vi "Pathing V2.vi"() -> ()   [LabVIEW 2017]
uses:
  <vilib>/robotics/Navigation/shared/WorldMap/OccupancyGridWorldMap/NI_Robotics_OccupancyGridWorldMap.lvclass
  040-typeDefs/Position.ctl
  <vilib>/Analysis/NI_AALPro.lvlib
panel:
  out "Numeric":i32=24
  in  "Position":T1={"X Pos"=300.0, "Y Pos"=0.0, "Bearing"=0.0}
  in  "Initialpos":cluster{dbl, dbl, dbl}={300.0, 0.0, 0.0}
  out "path":cluster{"X":i32, "Y":i32}[](array[cluster])=[{"X"=3, "Y"=0}, {"X"=3, "Y"=1}, {"X"=3, "Y"=2}, {"X"=3, "Y"=3}, {"X"=3, "Y"=4}, {"X"=3, "Y"=5}, {"X"=3, "Y"=6}]
  out "XY Graph 3":cluster{dbl[], dbl[]}(graph)={[0.0, 0.0, 0.0, 0.0, 0.0, 0.0], [100.0, 200.0, 300.0, 400.0, 500.0, 600.0]}
  in  "Robot Relative Position":cluster{"PosX":dbl, "PosY":dbl}={"PosX"=-300.0, "PosY"=50.0}
  in  "map reference in 2":refnum<data-value>
  in  "map reference in":refnum<data-value>
  in  "stop 2":bool
  out "output cluster":cluster{"PosX":dbl, "PosY":dbl}
  in  "Resolution":dbl=100.0
  out "Intensity Graph":dbl[][](graph)
  out "XY Graph 2":cluster{dbl[], dbl[]}(graph)
  out "Final X, Y, BEARING":cluster{dbl, dbl, dbl}={245.38756896666968, 124.45046063453532, -26.464846153846153}
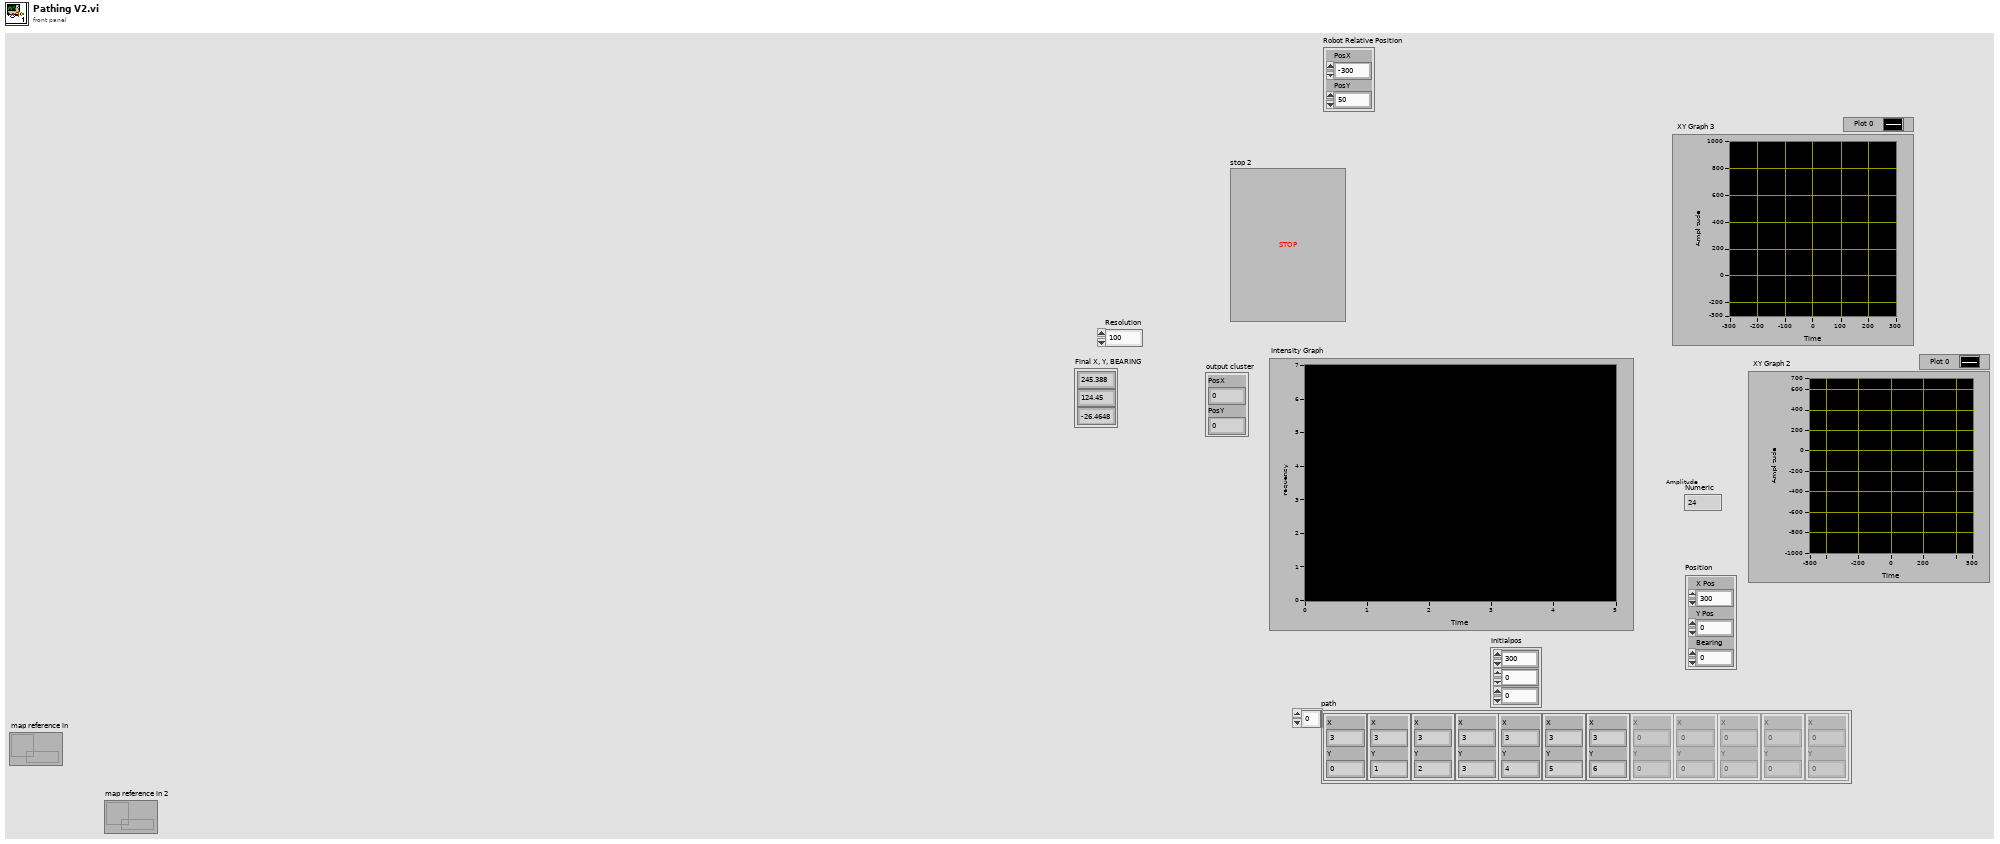
[diagram p1: front panel]
types:
  T1 = typedef "Position.ctl" = cluster{"X Pos":dbl, "Y Pos":dbl, "Bearing":dbl}
  T2 = typedef "LidarPoint.ctl" = cluster{"X":dbl, "Y":dbl}
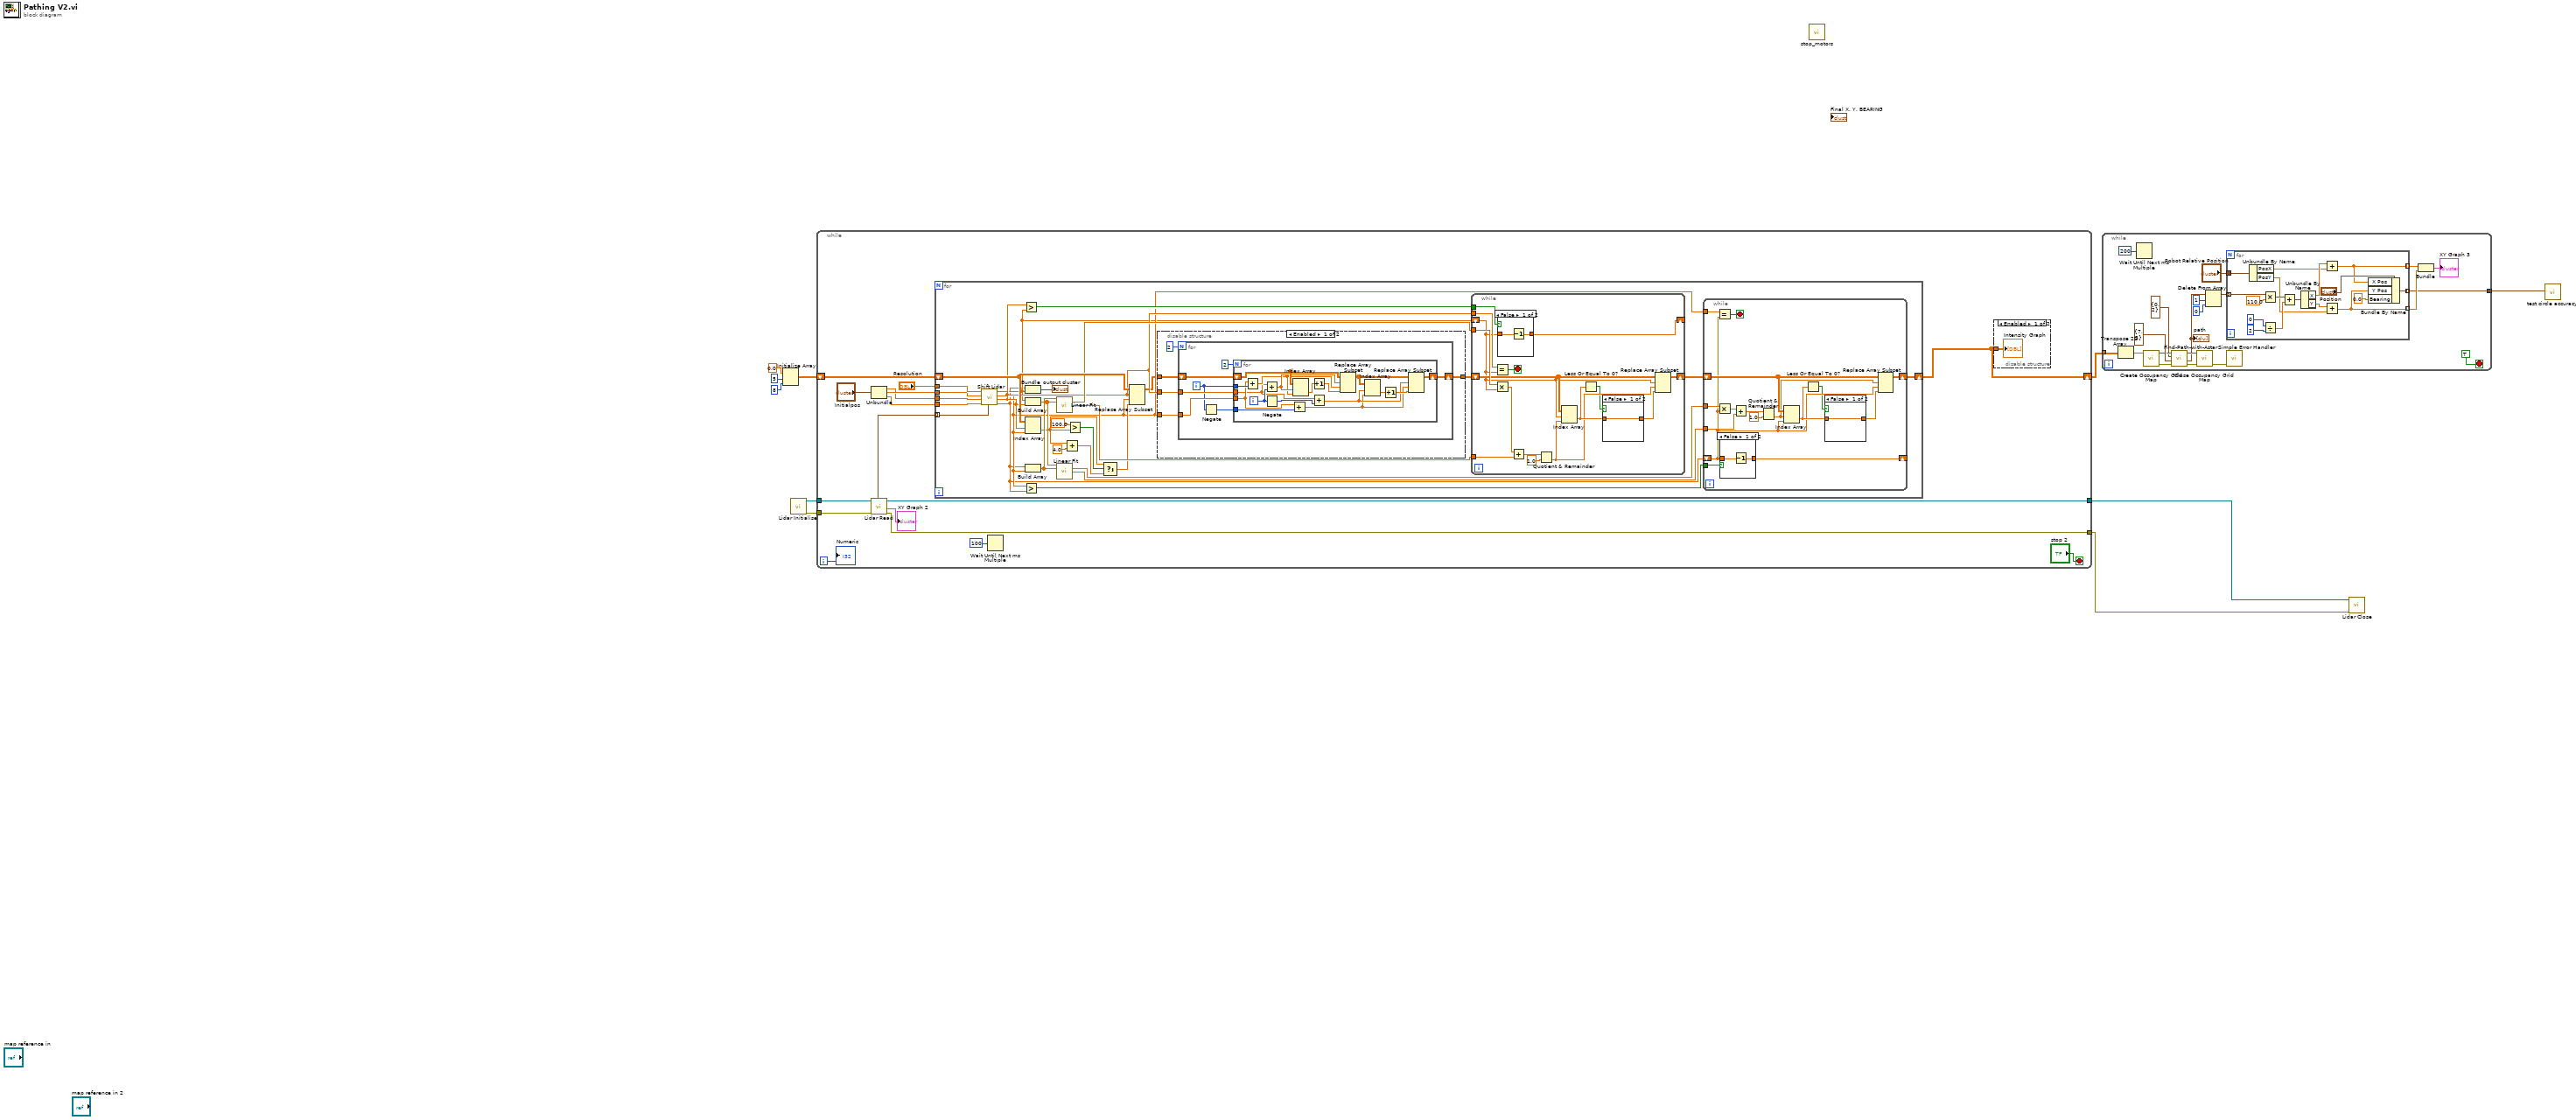
[diagram p0: block diagram]
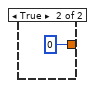
[diagram p4: hidden frame]
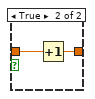
[diagram p5: hidden frame]
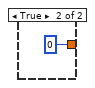
[diagram p6: hidden frame]
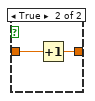
[diagram p7: hidden frame]
diagram:
  n1 = Initialize Array(0.0 ("element"), 5 ("dimension size"), 8 ("dimension size")) -> (w4:dbl[][])
  n2 = call "Lidar Initialise.vi"() -> ("error out"=w10:errorcluster, "VISA resource name out"=w3:refnum<visa-resource-name>)  [unwired: 10 in]
  n3 = while {
    tunnel: w3 -> [w26]
    tunnel: w10 -> [w25]
    tunnel: [w24] -> w9
    tunnel: [w23] -> w8
    shift-right: [w18] -> w2
    shift-left: w4 -> [w20]
    i -> [w11]
    stop <- "stop 2" stop-if-true
    n4 = Unbundle("Initialpos") -> (w13:dbl, w14:dbl, w12:dbl)
    n5 = call "Lidar Read.vi"("error in (no error)"=w25, "VISA resource name"=w26) -> ("error out"=w23:errorcluster, "Visual Out"=→"XY Graph 2":cluster{dbl[], dbl[]}, "VISA resource name out"=w24:refnum<visa-resource-name>, "XYflipped"=w19:T2[])  [unwired: 2 in, 3 out]
    n6 = for {
      tunnel: w14 -> [w54]
      tunnel: w13 -> [w49]
      tunnel: "Resolution" -> [w56]
      tunnel: w19 -> [w55] mode=indexing
      shift-right: [w34] -> w18
      shift-left: w20 -> [w53]
      tunnel: w12 -> [w33]
      n7 = call "Shift Lidar.vi"("XY"=w55, "Angle"=w33, "X position"=w49, "Y position"=w54, "Resolution"=w56) -> ("PosY"=w30:dbl, "Shifted X"=w36:dbl, "Shifted Y"=w35:dbl, "PosX"=w31:dbl)  [unwired: 3 in]
      n8 = Greater?(x=w36, y=w31) -> (0:w50:bool)
      n9 = Greater?(x=w35, y=w30) -> (0:w46:bool)
      n10 = Bundle("PosY"=w30, "PosX"=w31) -> (→"output cluster":cluster{"PosY":dbl, "PosX":dbl})  [unwired: 1 in]
      n11 = Build Array(w31, w36) -> (w44:dbl[])
      n12 = Index Array(array=w53, index (row)=w36, index (col)=w35) -> (element=w37:dbl)
      n13 = Build Array(w30, w35) -> (w45:dbl[])
      n14 = call <vilib>:"Linear Fit.vi"("Y"=w45, "X"=w44) -> ("slope"=w52:dbl, "intercept"=w51:dbl)  [unwired: 9 in, 3 out]
      n15 = call <vilib>:"Linear Fit.vi"("Y"=w44, "X"=w45) -> ("slope"=w43:dbl, "intercept"=w42:dbl)  [unwired: 9 in, 3 out]
      n16 = Add(x=w37, y=4.0) -> (x+y=w38:dbl)
      n17 = Greater?(x=100.0, y=w37) -> (0:w40:bool)
      n18 = Select(t=w37, s=w40, f=w38) -> (s? t:f=w41:dbl)
      n19 = Replace Array Subset(array=w53, new element=w41, index (row)=w36, index (col)=w35) -> (w29:dbl[][])
      n20 = disable-structure shown="Enabled" {
        disable-tunnel: w36 -> [w60 _]
        disable-tunnel: w35 -> [w59 _]
        disable-tunnel: w29 -> [w58 _]
        disable-tunnel: [w57 _] -> w28
        frame Enabled {
          n21 = for {
            N: 2 -> [_]
            tunnel: w60 -> [w66]
            tunnel: w59 -> [w64]
            shift-right: [w67] -> w57
            shift-left: w58 -> [w68]
            i -> [w63]
            n22 = Negate(x=w63) -> (-x=w62:i32)
            n23 = for {
              N: 2 -> [_]
              tunnel: w66 -> [w73]
              tunnel: w64 -> [w74]
              tunnel: w63 -> [w78]
              tunnel: w62 -> [w72]
              shift-right: [w81] -> w67
              shift-left: w68 -> [w83]
              i -> [w79]
              n24 = Add(x=w74, y=w78) -> (x+y=w75:dbl)
              n25 = Add(x=w73, y=w79) -> (x+y=w76:dbl)
              n26 = Negate(x=w79) -> (-x=w71:i32)
              n27 = Add(x=w74, y=w72) -> (x+y=w69:dbl)
              n28 = Index Array(array=w83, index (row)=w76, index (col)=w75) -> (element=w85:dbl)
              n29 = Increment(x=w85) -> (x+1=w77:dbl)
              n30 = Add(x=w73, y=w71) -> (x+y=w70:dbl)
              n31 = Replace Array Subset(array=w83, new element=w77, index (row)=w76, index (col)=w75) -> (w82:dbl[][])
              n32 = Index Array(array=w82, index (row)=w70, index (col)=w69) -> (element=w84:dbl)
              n33 = Increment(x=w84) -> (x+1=w80:dbl)
              n34 = Replace Array Subset(array=w82, new element=w80, index (row)=w70, index (col)=w69) -> (w81:dbl[][])
            }
          }
        }
        frame Disabled {
        }
      }
      n35 = while {
        tunnel: w36 -> [w122]
        shift-right: [w120] -> _
        shift-left: w31 -> [w115]
        tunnel: w52 -> [w119]
        tunnel: w51 -> [w117]
        tunnel: w50 -> [w121]
        shift-right: [w114] -> w47
        shift-left: w28 -> [w116]
        stop <- w123 stop-if-true
        n36 = Equal?(x=w122, y=w115) -> (x = y?=w123:bool)
        n37 = Multiply(x=w119, y=w115) -> (x*y=w118:dbl)
        n38 = case shown="False" w121 {
          tunnel: w115 -> [w126 w129]
          tunnel: [w127 w128] -> w120
          frame False {
            n39 = Decrement(x=w126) -> (x-1=w127:dbl)
          }
          frame True {
            n40 = Increment(x=w129) -> (x+1=w128:dbl)
          }
        }
        n41 = Add(x=w118, y=w117) -> (x+y=w111:dbl)
        n42 = Quotient & Remainder(x=w111, y=1.0) -> (floor(x/y)=w109:dbl)  [unwired: 1 out]
        n43 = Index Array(array=w116, index (row)=w115, index (col)=w109) -> (element=w112:dbl)
        n44 = Less Or Equal To 0?(x=w112) -> (x <= 0?=w108:bool)
        n45 = case shown="False" w108 {
          tunnel: [w124 0] -> w113
          tunnel: w112 -> [w124 _]
          frame False {
          }
          frame True {
          }
        }
        n46 = Replace Array Subset(array=w116, new element=w113, index (row)=w115, index (col)=w109) -> (w114:dbl[][])
      }
      n47 = while {
        shift-right: [w91] -> w34
        shift-left: w47 -> [w90]
        shift-right: [w98] -> _
        shift-left: w30 -> [w88]
        tunnel: w35 -> [w100]
        tunnel: w46 -> [w99]
        tunnel: w43 -> [w97]
        tunnel: w42 -> [w95]
        stop <- w101 stop-if-true
        n48 = Equal?(x=w100, y=w88) -> (x = y?=w101:bool)
        n49 = Multiply(x=w97, y=w88) -> (x*y=w96:dbl)
        n50 = case shown="False" w99 {
          tunnel: w88 -> [w104 w107]
          tunnel: [w105 w106] -> w98
          frame False {
            n51 = Decrement(x=w104) -> (x-1=w105:dbl)
          }
          frame True {
            n52 = Increment(x=w107) -> (x+1=w106:dbl)
          }
        }
        n53 = Add(x=w96, y=w95) -> (x+y=w94:dbl)
        n54 = Quotient & Remainder(x=w94, y=1.0) -> (floor(x/y)=w87:dbl)  [unwired: 1 out]
        n55 = Index Array(array=w90, index (row)=w87, index (col)=w88) -> (element=w92:dbl)
        n56 = Less Or Equal To 0?(x=w92) -> (x <= 0?=w86:bool)
        n57 = case shown="False" w86 {
          tunnel: [w102 0] -> w89
          tunnel: w92 -> [w102 _]
          frame False {
          }
          frame True {
          }
        }
        n58 = Replace Array Subset(array=w90, new element=w89, index (row)=w87, index (col)=w88) -> (w91:dbl[][])
      }
    }
    n59 = Wait Until Next ms Multiple(millisecond multiple=u32 100) -> ()  [unwired: 1 out]
    n60 = disable-structure shown="Enabled" {
      disable-tunnel: w18 -> [w27 _]
      frame Enabled {
        "Intensity Graph" <- w27
      }
      frame Disabled {
      }
    }
    "Numeric" <- w11
  }
  n61 = call "stop_motors.vi"() -> ()  [unwired: 5 in, 1 out]
  n62 = while {
    tunnel: w2 -> [w135]
    tunnel: [w130] -> w1
    stop <- TRUE stop-if-true
    n63 = Transpose 2D Array(2D array=w135) -> (transposed array=w143:dbl[][])
    n64 = Wait Until Next ms Multiple(millisecond multiple=u32 200) -> ()  [unwired: 1 out]
    n65 = call <vilib>:"Create Occupancy Grid Map.vi"("occupancy grid"=w143) -> ("error out"=w144:errorcluster, "map reference out"=w145:refnum<data-value>)  [unwired: 9 in]
    n66 = call "Find-Path-with-Astar.vi"("error in (no error)"=w144, "goal node"=cluster{"x":i32, "y":i32} {"x"=7, "y"=2} ("endPos"), "start node"=cluster{"x":i32, "y":i32} {"x"=0, "y"=2} ("t"), "map reference in"=w145) -> ("error out"=w148:errorcluster, "Array"=w139:cluster{"X":i32, "Y":i32}[], "map reference out"=w149:refnum<data-value>)  [unwired: 5 in]
    "path" <- w139
    n67 = call <vilib>:"Close Occupancy Grid Map.vi"("error in (no error)"=w148, "map reference in"=w149) -> ("error out"=w147:errorcluster)  [unwired: 9 in]
    n68 = Delete From Array(array=w139, length=1, index=0) -> (array with subset deleted=w140:cluster{"X":i32, "Y":i32}[])  [unwired: 1 out]
    n69 = for {
      tunnel: w140 -> [w160] mode=indexing
      tunnel: "Robot Relative Position" -> [w166]
      tunnel: [w152] -> w130 mode=indexing
      tunnel: [w151] -> w132 mode=indexing
      tunnel: [w150] -> w131 mode=indexing
      n70 = Unbundle By Name(w166) -> ("PosX"=w157:dbl, "PosY"=w155:dbl)
      n71 = Multiply(x=w160, y=110.0) -> (x*y=w164:cluster{"X":dbl, "Y":dbl})
      n72 = Divide(x=0, y=2) -> (x/y=w165:dbl)
      n73 = Add(x=w164, y=w165) -> (x+y=w159:cluster{"X":dbl, "Y":dbl})
      n74 = Unbundle By Name(w159) -> ("X"=w158:dbl, "Y"=w156:dbl)
      n75 = Add(x=w158, y=w157) -> (x+y=w151:dbl)
      n76 = Add(x=w156, y=w155) -> (x+y=w150:dbl)
      n77 = Bundle By Name(cluster="Position", "X Pos"=w151, "Y Pos"=w150, "Bearing"=0.0) -> (w152:T1)
    }
    n78 = call <vilib>:"Simple Error Handler.vi"("error in (no error)"=w147) -> ()  [unwired: 4 in, 5 out]
    n79 = Bundle(w132, w131) -> (→"XY Graph 3":cluster{dbl[], dbl[]})  [unwired: 1 in]
  }
  n80 = call "Lidar Close.vi"("error in (no error)"=w8, "VISA resource name"=w9) -> ()  [unwired: 9 in, 1 out]
  n81 = call "test circle accuracy.vi"("Array of Points"=w1) -> ()  [unwired: 11 in]
